vi "Draw.vi"(8 "error in (no error)":errorcluster, 11 "Grid in":refnum<class "Grid.lvclass">) -> (0 "error out":errorcluster, 2 "Picture":picture, 3 "Grid out":refnum<class "Grid.lvclass">)   [LabVIEW 2017, in "LV Image Editor Framework.lvlib" / "Grid.lvclass"]
uses:
  <vilib>/LIEF/Forms/Grid/Grid.lvclass
  <vilib>/LIEF/Forms/Grid/Grid.lvclass/Grid.ctl
  <vilib>/LIEF/Forms/Line/Line.lvclass
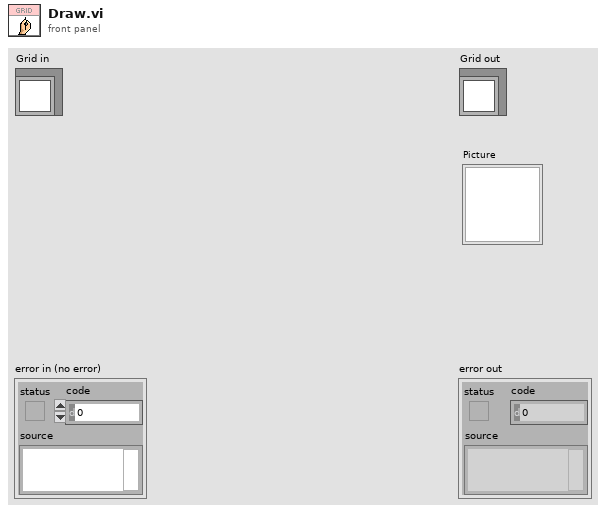
[diagram p1: front panel]
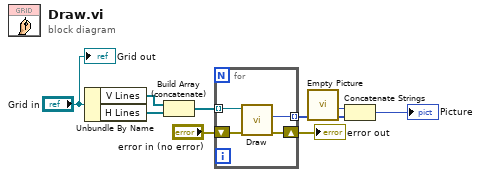
[diagram p0: block diagram]
diagram:
  n1 = Unbundle By Name("Grid in") -> ("V Lines"=w9:refnum<class "Line.lvclass">[], "H Lines"=w8:refnum<class "Line.lvclass">[])
  n2 = Build Array (concatenate)(w9, w8) -> (w7:refnum<class "Line.lvclass">[])
  n3 = for {
    tunnel: w7 -> [w13] mode=indexing
    tunnel: [w12] -> w5 mode=indexing
    shift-right: [w11] -> w2
    shift-left: "error in (no error)" -> [w10]
    n4 = call-dynamic "Draw.vi"("error in (no error)"=w10, "Line in"=w13) -> ("error out"=w11:errorcluster, "Picture"=w12:picture)  [unwired: 7 in, 1 out]
  }
  "error out" <- w2
  n5 = call "Empty Picture"() -> ("empty picture"=w4:picture)
  n6 = Concatenate Strings(w4, w5) -> (→"Picture":picture)
  "Grid out" <- "Grid in"
